vi "test_refnumProject.vi"(8 "error in (no error)":errorcluster) -> (0 "error out":errorcluster)   [LabVIEW 2013]
uses:
  run-tests/Run Test (ProjectRefnum).vi
  Caraya.lvlib
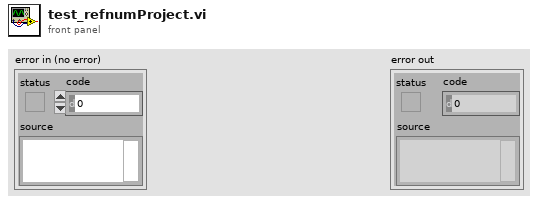
[diagram p1: front panel]
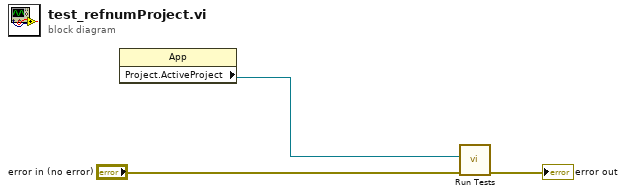
[diagram p0: block diagram]
diagram:
  n1 = property class="App"() -> ("Project.ActiveProject"=w1:refnum<vi>)  [unwired: 2 in, 2 out]
  n2 = call-poly "Run Tests.vi"("error in"="error in (no error)", "Project Refnum"=w1) -> ("error out"=→"error out":errorcluster)  [unwired: 9 in]
